vi "Phasor Explorer Queue.vi"(10 "create if not found? (F)":bool) -> (2 "Phasor Explorer Queue":refnum<queue>)   [LabVIEW 2019]
uses:
  Phasor Explorer Q [Element].ctl
  Phasor Explorer Q [Event] List.ctl
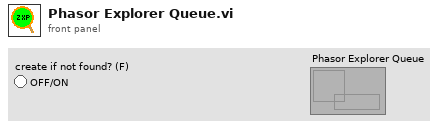
[diagram p1: front panel]
types:
  T1 = typedef "Phasor Explorer Q [Element].ctl" = cluster{"ZXP Q Event":T2, "Data":variant}
  T2 = typedef "Phasor Explorer Q [Event] List.ctl" = enum16{"Idle", "Initialization", "Show-Hide UC Ticks", "Edit User-defined Gate/IRF", "Update Phasor Graph", "Update Sum of Gates Graph", "Update Parameters", "Compute Decay &/or Gates", "Find Pseudo UC Intersections", "Compute alpha(beta) Plot", "Compute Pseudo-Phase Lifetime Plot", "Export Parameters to Clipboard", "Update Phase & Modulus Lifetime", "XY Graph Special Event", "Update Graph Plots Info", "Fit to Circle", "Quit"}
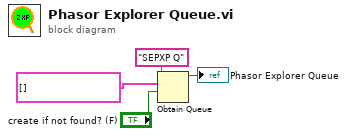
[diagram p0: block diagram]
diagram:
  n1 = Obtain Queue(name (unnamed)="SEPXP Q", element data type=T1[] [] ("PSEXP Q Element"), create if not found? (T)="create if not found? (F)") -> (queue out=→"Phasor Explorer Queue":refnum<queue>)  [unwired: 2 in, 2 out]
